vi "HeaderAction.vi"(0 "InstrClass":refnum<class "SymphonyCCD.lvclass"> caption="DNL_LabVIEW Object in", 11 "error in (no error)":errorcluster caption="entrée d'erreur (pas d'erreur)") -> (4 "InstrClassOut":refnum<class "SymphonyCCD.lvclass"> caption="DNL_LabVIEW Object out", 6 "DataNames":string[](array[string]), 8 "Instr Name":string, 10 "HeaderString":string, 13 "ArrDisplayNames":string[](array[string]), 14 "DisplayNames":string[](array[string]), 15 "error out":errorcluster caption="sortie d'erreur")   [LabVIEW 2019, in "SymphonyCCD.lvclass"]
uses:
  SymphonyCCD.lvclass
  C:/Programmes Labview/LabScanV1A/DevicesClass/BaseDevice/BaseDevice.lvclass
  <userlib>/JY Symphony/NoiseCorr.ctl
  SymphonyCCD.lvclass/SymphonyCCD.ctl
  <userlib>/GenProg/ReadValByRefU32.vi
  <userlib>/GenProg/ReadValByRefDbl.vi
  <userlib>/GenProg/ReadValByRefBool.vi
  BaseDevice/BaseDevice.lvclass
panel:
  in  "Noise Mode":T1=enum."One For All Acq"
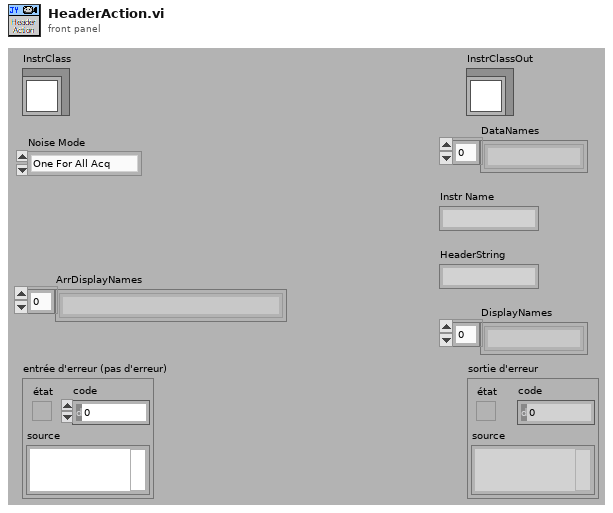
[diagram p1: front panel]
types:
  T1 = typedef "NoiseCorr.ctl" = enum16{"Off", "One For All Acq", "One For Every Acq"}
  T2 = typedef "SymphonyCCD.lvclass/SymphonyCCD_Func.ctl" = enum16{"AcqImageSim (Counts)", "AcqImage (Counts)"}
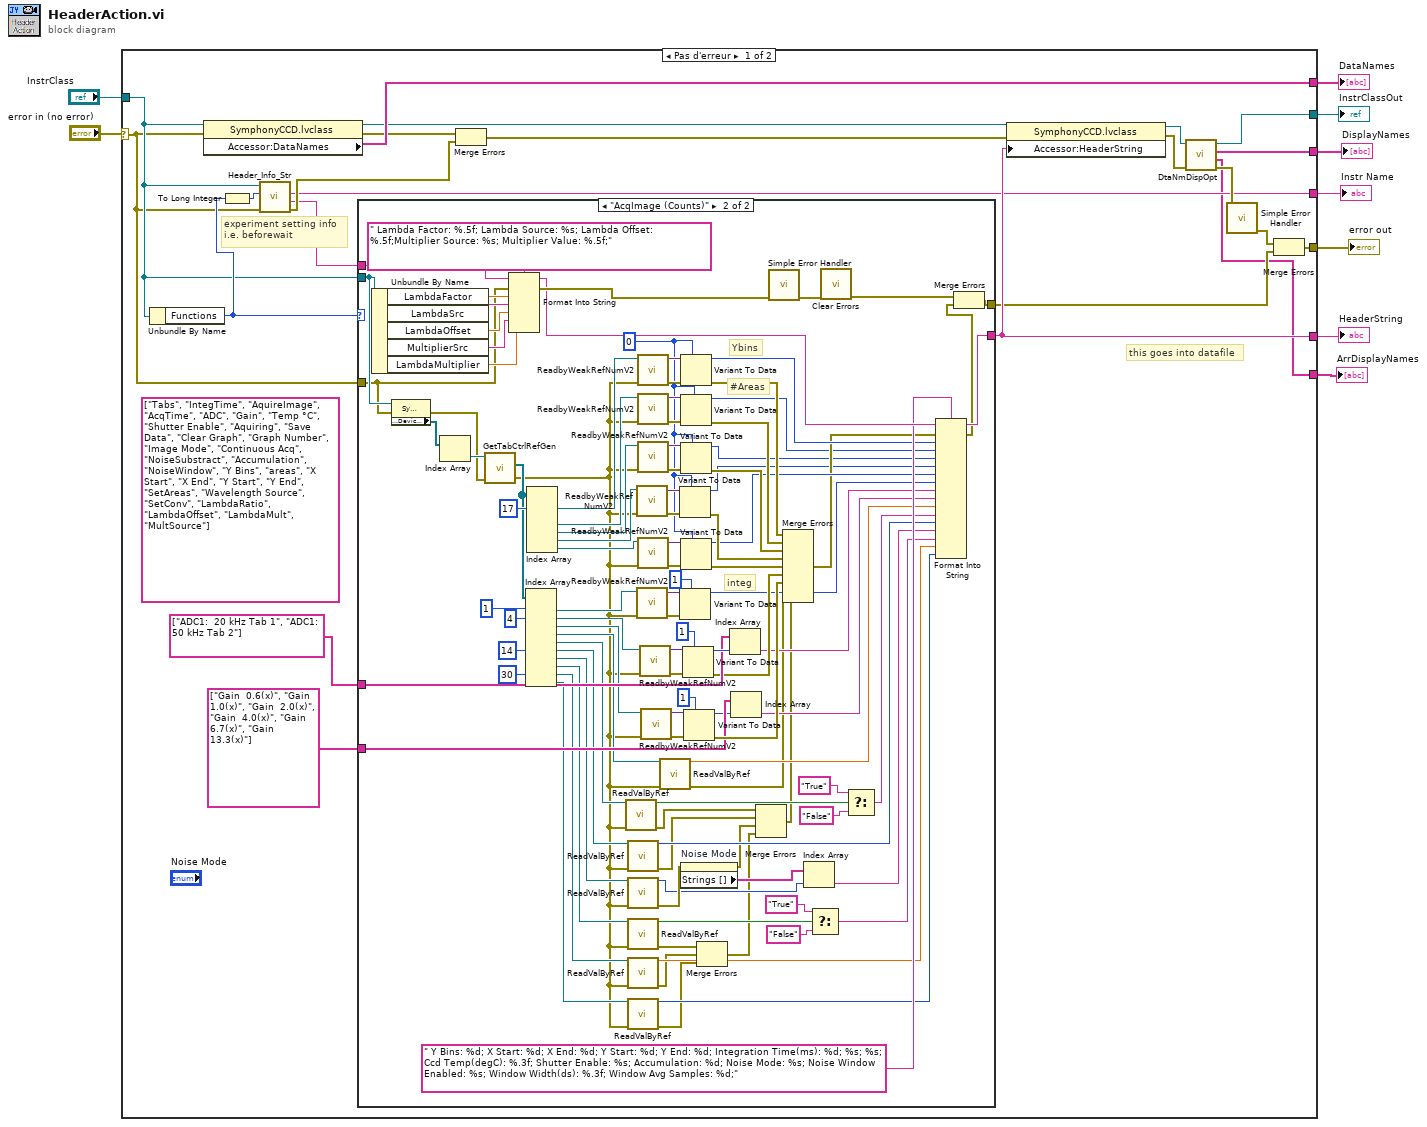
[diagram p0: block diagram]
diagram:
  n1 = case shown="Pas d'erreur" "error in (no error)" {
    selector: "error in (no error)" -> [w16 w141]
    tunnel: [w29 _] -> w8
    tunnel: [w32 _] -> w7
    tunnel: "InstrClass" -> [w17 w142]
    tunnel: [w14 w141] -> w5
    tunnel: [w26 w142] -> w3
    tunnel: [w20 _] -> w4
    tunnel: [w24 _] -> w2
    tunnel: [w10 _] -> w1
    frame No Error {
      (unwired) string[] ["Tabs", "IntegTime", "AquireImage", "AcqTime", "ADC", "Gain", "Temp °C", "Shutter Enable", "Aquiring", "Save Data", "Clear Graph", "Graph Number", "Image Mode", "Continuous Acq", "NoiseSubstract", "Accumulation", "NoiseWindow", "Y Bins", "areas", "X Start", "X End", "Y Start", "Y End", "SetAreas", "Wavelength Source", "SetConv", "LambdaRatio", "LambdaOffset", "LambdaMult", "MultSource"] ("ControlsNames")
      # "this goes into datafile"
      # "experiment setting info\ni.e. beforewait"
      n2 = Unbundle By Name(w17) -> ("Functions"=w18:T2)
      n3 = property class="SymphonyCCD.lvclass"(reference=w17, error in=w16) -> (reference out=w31:refnum<class "SymphonyCCD.lvclass">, error out=w30:errorcluster, "Accessor:DataNames"=w32:string[])
      n4 = To Long Integer(number=w18) -> (32bit integer=w19:i32)
      n5 = call-dynamic "Header_Info_Str.vi"("error in (no error)"=w16, "Functions"=w19, "DefaultDev in"=w17) -> ("error out"=w22:errorcluster, "HdrInfoStr"=w21:string, "InstrumentName"=w20:string)  [unwired: 5 in, 1 out]
      n6 = case shown="\"AcqImage (Counts)\"" w18 {
        tunnel: [w33 w122] -> w29
        tunnel: w21 -> [w33 w137]
        tunnel: w17 -> [_ w130]
        tunnel: w16 -> [_ w127]
        tunnel: [_ w125] -> w13
        tunnel: string[] ["ADC1:  20 kHz Tab 1", "ADC1:  50 kHz Tab 2"] ("ControlsNames") -> [_ w82]
        tunnel: string[] ["Gain  0.6(x)", "Gain  1.0(x)", "Gain  2.0(x)", "Gain  4.0(x)", "Gain  6.7(x)", "Gain 13.3(x)"] ("Strings []") -> [_ w75]
        frame Default {
        }
        frame "AcqImage (Counts)" {
          w108 = 0
          # "integ"
          # "#Areas"
          # "Ybins"
          n7 = Unbundle By Name(w130) -> ("LambdaFactor"=w140:dbl, "LambdaSrc"=w138:string, "LambdaOffset"=w139:dbl, "MultiplierSrc"=w132:string, "LambdaMultiplier"=w131:dbl)
          n8 = property class="SymphonyCCD.lvclass"(reference=w130, error in=w127) -> (error out=w126:errorcluster, "Accessor:DeviceCtrl"=w129:refnum<vi>[])  [unwired: 1 out]
          n9 = Index Array(array=w129) -> (element=w128:refnum<vi>)  [unwired: 1 in]
          n10 = call <userlib>:"GetTabCtrlRefGen.vi"("ErrorIn(No Error)"=w126, "CommandRef"=w128) -> ("sortie d'erreur"=w40:errorcluster, "ControlsRefs"=w91:refnum<vi>[])  [unwired: 7 in, 1 out]
          n11 = Format Into String(format string=" Lambda Factor: %.5f; Lambda Source: %s; Lambda Offset: %.5f;Multiplier Source: %s; Multiplier Value: %.5f;", initial string=w137, error in=w127, w140, w138, w139, w132, w131) -> (resulting string=w123:string, error out=w135:errorcluster)
          n12 = Index Array(array=w91, index #1=1 ("index"), index #2=4 ("index"), index #6=14 ("index"), index #9=30 ("index")) -> (element #1=w87:refnum<vi>, element #2=w79:refnum<vi>, element #3=w70:refnum<vi>, element #4=w69:refnum<vi>, element #5=w66:refnum<vi>, element #6=w57:refnum<vi>, element #7=w55:refnum<vi>, element #8=w54:refnum<vi>, element #9=w42:refnum<vi>, element #10=w41:refnum<vi>)  [unwired: 6 in]
          n13 = Index Array(array=w91, index #1=17 ("index")) -> (element #1=w120:refnum<vi>, element #3=w113:refnum<vi>, element #4=w95:refnum<vi>, element #5=w94:refnum<vi>, element #6=w93:refnum<vi>)  [unwired: 5 in, 1 out]
          n14 = call-poly <userlib>:"ReadValByRef.vi"("Control Ref"=w66, "error in"=w40) -> ("Valeur"=w60:bool, "error out"=w52:errorcluster)  [unwired: 12 in]
          n15 = call-poly <userlib>:"ReadValByRef.vi"("Control Ref"=w57, "error in"=w40) -> ("Valeur"=w56:u32, "error out"=w51:errorcluster)  [unwired: 12 in]
          n16 = call-poly <userlib>:"ReadValByRef.vi"("Control Ref"=w55, "error in"=w40) -> ("Valeur"=w46:u32, "error out"=w48:errorcluster)  [unwired: 12 in]
          n17 = call-poly <userlib>:"ReadValByRef.vi"("Control Ref"=w54, "error in"=w40) -> ("Valeur"=w53:bool, "error out"=w37:errorcluster)  [unwired: 12 in]
          n18 = call-poly <userlib>:"ReadValByRef.vi"("Control Ref"=w42, "error in"=w40) -> ("Valeur"=w39:dbl, "error out"=w36:errorcluster)  [unwired: 12 in]
          n19 = call-poly <userlib>:"ReadValByRef.vi"("Control Ref"=w41, "error in"=w40) -> ("Valeur"=w38:u32, "error out"=w35:errorcluster)  [unwired: 12 in]
          n20 = call <userlib>:"ReadbyWeakRefNumV2.vi"("error in"=w40, "Control Ref"=w94) -> ("error out"=w112:errorcluster, "Valeur"=w109:variant)  [unwired: 8 in]
          n21 = call <userlib>:"ReadbyWeakRefNumV2.vi"("error in"=w40, "Control Ref"=w87) -> ("error out"=w92:errorcluster, "Valeur"=w65:variant)  [unwired: 8 in]
          n22 = call <userlib>:"ReadbyWeakRefNumV2.vi"("error in"=w40, "Control Ref"=w120) -> ("error out"=w114:errorcluster, "Valeur"=w115:variant)  [unwired: 8 in]
          n23 = call <userlib>:"ReadbyWeakRefNumV2.vi"("error in"=w40, "Control Ref"=w113) -> ("error out"=w116:errorcluster, "Valeur"=w117:variant)  [unwired: 8 in]
          n24 = call <userlib>:"ReadbyWeakRefNumV2.vi"("error in"=w40, "Control Ref"=w95) -> ("error out"=w119:errorcluster, "Valeur"=w118:variant)  [unwired: 8 in]
          n25 = call <userlib>:"ReadbyWeakRefNumV2.vi"("error in"=w40, "Control Ref"=w93) -> ("error out"=w111:errorcluster, "Valeur"=w110:variant)  [unwired: 8 in]
          n26 = call <userlib>:"ReadbyWeakRefNumV2.vi"("error in"=w40, "Control Ref"=w79) -> ("error out"=w89:errorcluster, "Valeur"=w84:variant)  [unwired: 8 in]
          n27 = call <userlib>:"ReadbyWeakRefNumV2.vi"("error in"=w40, "Control Ref"=w70) -> ("error out"=w78:errorcluster, "Valeur"=w81:variant)  [unwired: 8 in]
          n28 = call-poly <userlib>:"ReadValByRef.vi"("Control Ref"=w69, "error in"=w40) -> ("Valeur"=w68:dbl, "error out"=w67:errorcluster)  [unwired: 12 in]
          n29 = Variant To Data(error in=w112, type=w108, Variant=w109) -> (data=w98:i32, error out=w104:errorcluster)
          n30 = Variant To Data(error in=w92, type=u32 1 ("index"), Variant=w65) -> (data=w71:u32)  [unwired: 1 out]
          n31 = Variant To Data(error in=w114, type=w108, Variant=w115) -> (data=w107:i32, error out=w101:errorcluster)
          n32 = Variant To Data(error in=w116, type=w108, Variant=w117) -> (data=w96:i32, error out=w102:errorcluster)
          n33 = Variant To Data(error in=w119, type=w108, Variant=w118) -> (data=w97:i32, error out=w103:errorcluster)
          n34 = Variant To Data(error in=w111, type=w108, Variant=w110) -> (data=w100:i32, error out=w105:errorcluster)
          n35 = property on="Noise Mode" class="Énum (strict)"(error in=w48) -> (error out=w47:errorcluster, "Strings []"=w49:string[])  [unwired: 1 in, 1 out]
          n36 = Variant To Data(error in=w89, type=u16 1 ("index"), Variant=w84) -> (data=w83:u16, error out=w77:errorcluster)
          n37 = Variant To Data(error in=w78, type=u16 1 ("index"), Variant=w81) -> (data=w74:u16, error out=w76:errorcluster)
          n38 = Merge Errors(w37, w36, w35) -> (w34:errorcluster)
          n39 = Index Array(array=w82, index=w83) -> (element=w73:string)
          n40 = Index Array(array=w75, index=w74) -> (element=w72:string)
          n41 = Merge Errors(w52, w51, w47, w34) -> (w50:errorcluster)
          n42 = call <vilib>:"Simple Error Handler.vi"("error in (no error)"=w135) -> ("error out"=w134:errorcluster)  [unwired: 4 in, 4 out]
          n43 = Merge Errors(w101, w102, w103, w104, w105, w77, w76, w67, w50) -> (w99:errorcluster)
          n44 = Index Array(array=w49, index=w46) -> (element=w45:string)
          n45 = Select(t="True", s=w53, f="False") -> (s? t:f=w44:string)
          n46 = call <vilib>:"Clear Errors.vi"("error in (no error)"=w134) -> ("error out"=w133:errorcluster)  [unwired: 5 in, 1 out]
          n47 = Select(t="True", s=w60, f="False") -> (s? t:f=w59:string)
          n48 = Format Into String(format string=" Y Bins: %d; X Start: %d; X End: %d; Y Start: %d; Y End: %d; Integration Time(ms): %d; %s; %s; Ccd Temp(degC): %.3f; Shutter Enable: %s; Accumulation: %d; Noise Mode: %s; Noise Window Enabled: %s; Window Width(ds): %.3f; Window Avg Samples: %d;", initial string=w123, error in=w99, w107, w96, w97, w98, w100, w71, w73, w72, w68, w59, w56, w45, w44, w39, w38) -> (resulting string=w122:string, error out=w106:errorcluster)
          n49 = Merge Errors(w133, w106) -> (w125:errorcluster)
        }
      }
      n50 = Merge Errors(w30, w22) -> (w23:errorcluster)
      n51 = property class="SymphonyCCD.lvclass"(reference=w31, error in=w23, "Accessor:HeaderString"=w29) -> (reference out=w25:refnum<class "SymphonyCCD.lvclass">, error out=w28:errorcluster)
      n52 = call "DtaNmDispOpt.vi"("error in (no error)"=w28, "BaseDevice en entrée"=w25) -> ("error out"=w27:errorcluster, "ArrDisplayNames"=w10:string[], "DisplayNames"=w24:string[], "BaseDevice en sortie"=w26:refnum<class "SymphonyCCD.lvclass">)  [unwired: 6 in]
      n53 = call <vilib>:"Simple Error Handler.vi"("error in (no error)"=w27) -> ("error out"=w15:errorcluster)  [unwired: 4 in, 4 out]
      n54 = Merge Errors(w15, w13) -> (w14:errorcluster)
    }
    frame Error {
    }
  }
  "error out" <- w5
  "InstrClassOut" <- w3
  "DataNames" <- w7
  "HeaderString" <- w8
  "Instr Name" <- w4
  "DisplayNames" <- w2
  "ArrDisplayNames" <- w1
